vi "SetParam.vi"(8 "error in (no error)":errorcluster caption="entrée d'erreur (pas d'erreur)", 10 "make_low_rank_matrix":T1={"n_samples"=100, "n_features"=100, "effective_rank"=10, "tail_strength"=0.5, "random_state"=-1} {"random_state" min=-1; "tail_strength" min=0.0 max=1.0; "n_features" min=1; "n_samples" min=1}, 11 "Low_Rank_Matrix.lvclass":refnum<class "Low_Rank_Matrix.lvclass">) -> (0 "error out":errorcluster caption="sortie d'erreur", 3 "Low_Rank_Matrix.lvclass":refnum<class "Low_Rank_Matrix.lvclass">)   [LabVIEW 2020, in "Low_Rank_Matrix.lvclass"]
doc: "Set Parameters"
uses:
  Low_Rank_Matrix.lvclass
  Low_Rank_Matrix.lvclass/Low_Rank_Matrix.ctl
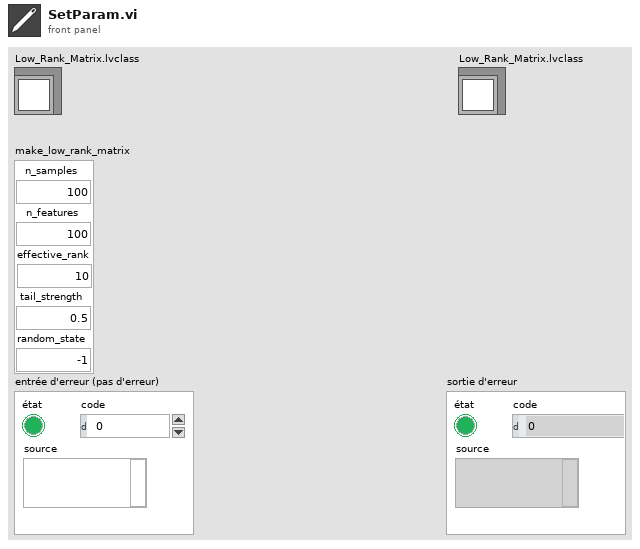
[diagram p1: front panel]
types:
  T1 = cluster{"n_samples":u32, "n_features":u32, "effective_rank":i32, "tail_strength":dbl, "random_state":i32}
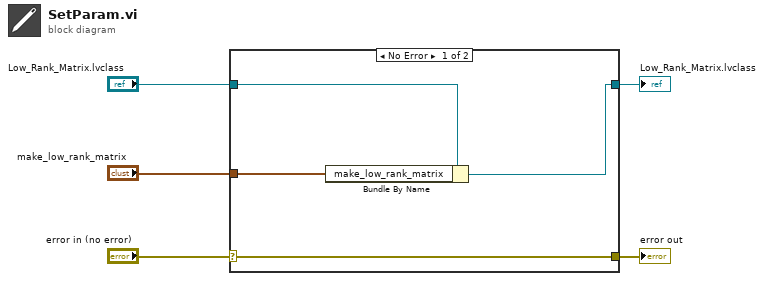
[diagram p0: block diagram]
diagram:
  n1 = case shown="No Error" "error in (no error)" {
    selector: "error in (no error)" -> [w9 w10]
    tunnel: [w9 w10] -> w4
    tunnel: [w7 w11] -> w2
    tunnel: "Low_Rank_Matrix.lvclass" -> [w8 w11]
    tunnel: "make_low_rank_matrix" -> [w6 _]
    frame No Error {
      n2 = Bundle By Name(cluster=w8, "make_low_rank_matrix"=w6) -> (w7:refnum<class "Low_Rank_Matrix.lvclass">)
    }
    frame Error {
    }
  }
  "error out" <- w4
  "Low_Rank_Matrix.lvclass" <- w2
